vi "gameOver.vi"(8 "error in (no error)":errorcluster, 11 "Simon_Game in":refnum<class "Simon_Game.lvclass">) -> (0 "error out":errorcluster, 3 "Simon_Game out":refnum<class "Simon_Game.lvclass">)   [LabVIEW 2019, in "Simon_Game.lvclass"]
uses:
  Simon_Game.lvclass
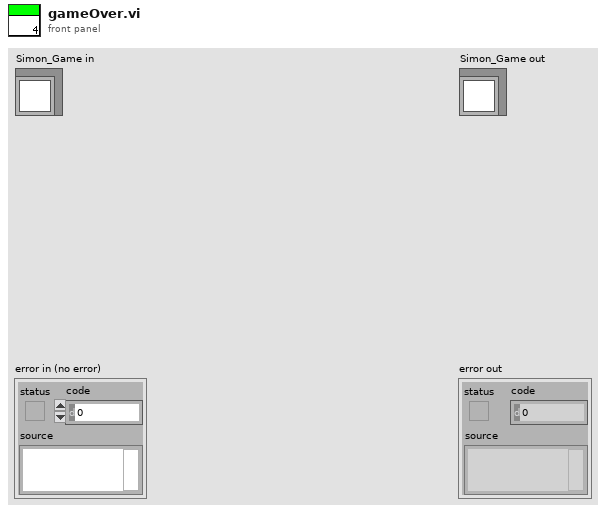
[diagram p1: front panel]
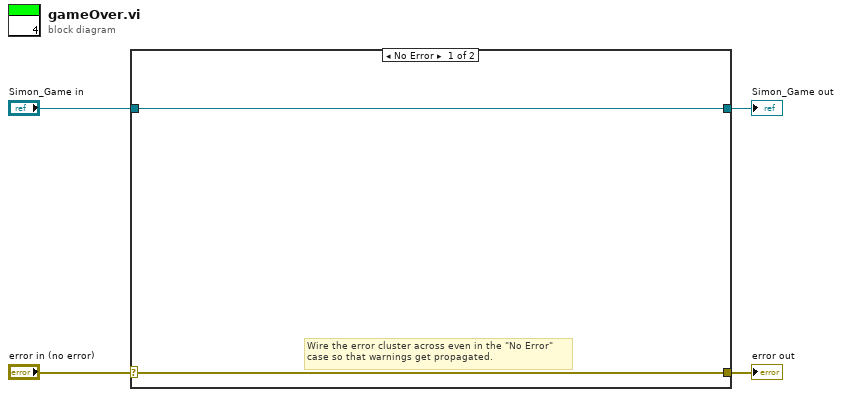
[diagram p0: block diagram]
diagram:
  n1 = case shown="No Error" "error in (no error)" {
    selector: "error in (no error)" -> [w5 w8]
    tunnel: [w5 w8] -> w3
    tunnel: [w6 w7] -> w1
    tunnel: "Simon_Game in" -> [w6 w7]
    frame No Error {
      # "Wire the error cluster across even in the \"No Error\"\ncase so that warnings get propagated."
    }
    frame Error {
    }
  }
  "error out" <- w3
  "Simon_Game out" <- w1
